vi "dfd_Sort Zeros in.vi"(11 "zeros in":cdb[](array[numeric])) -> (2 "another half":cdb[](array[numeric]), 3 "half zeros":cdb[](array[numeric]))   [LabVIEW 2017, in "NI_DigFilter_Design.lvlib"]
uses:
  <vilib>/addons/Digital Filter Design/NI_DigFilter_Design.lvlib
  <vilib>/addons/Digital Filter Design/StructCvt.llb/dfd_Get Alternate Components of Array (Real).vi
  <vilib>/addons/Digital Filter Design/NI_DigFilterLicensed.lvlib
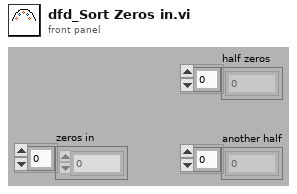
[diagram p1: front panel]
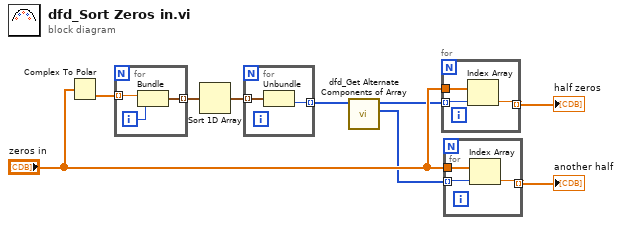
[diagram p0: block diagram]
diagram:
  n1 = Complex To Polar(r * e^(i*theta)="zeros in") -> (theta=w9:dbl[])  [unwired: 1 out]
  n2 = for {
    tunnel: w9 -> [w11] mode=indexing
    tunnel: [w10] -> w8 mode=indexing
    i -> [w12]
    n3 = Bundle(w11, w12) -> (w10:cluster{dbl, i32})  [unwired: 1 out]
  }
  n4 = Sort 1D Array(array=w8) -> (sorted array=w7:cluster{dbl, i32}[])
  n5 = for {
    tunnel: w7 -> [w14] mode=indexing
    tunnel: [w13] -> w3 mode=indexing
    n6 = Unbundle(w14) -> (w13:i32)  [unwired: 1 out]
  }
  n7 = call-poly <vilib>:"dfd_Get Alternate Components of Array.vi"("input array"=w3) -> ("another half"=w1:i32[], "half array"=w2:i32[])  [unwired: 9 out]
  n8 = for {
    tunnel: "zeros in" -> [w17]
    tunnel: [w16] -> w6 mode=indexing
    tunnel: w2 -> [w15] mode=indexing
    n9 = Index Array(array=w17, index=w15) -> (element=w16:cdb)
  }
  "half zeros" <- w6
  n10 = for {
    tunnel: "zeros in" -> [w20]
    tunnel: [w19] -> w5 mode=indexing
    tunnel: w1 -> [w18] mode=indexing
    n11 = Index Array(array=w20, index=w18) -> (element=w19:cdb)
  }
  "another half" <- w5
